vi "Touch and Limit controller.vi"(3 "error in (no error)":errorcluster) -> (0 "error out":errorcluster={"status"=TRUE, "code"=1172, "source"="Error calling method Aerotech.A3200.LabVIEW.DiagPacketPoller.Retrieve, (System.Reflection.TargetInvocationException: Exception has been thrown by the target of an invocation.\n\tInner Exception: System.NullReferenceException: Object reference not set to an instance of an object.) <append><b>System.NullReferenceException</b> in RetrieveDiagPacket.vi->Faults and Position data.vi->Aerotech Controller (main).vi"}, 1 "Limit Reached":bool, 2 "Touching":bool)   [LabVIEW 2011]
uses:
  <vilib>/DAQmx/read.llb/DAQmx Read (Digital Bool 1Line 1Point).vi
  <vilib>/DAQmx/create/channels.llb/DAQmx Create Channel (DI-Digital Input).vi
  <vilib>/DAQmx/miscellaneous.llb/DAQmx Fill In Error Info.vi
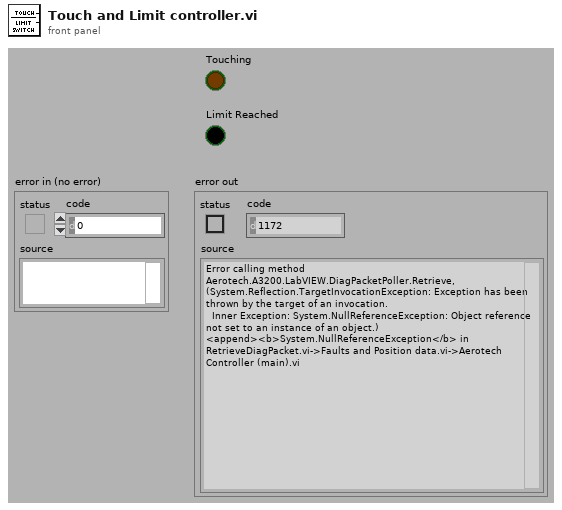
[diagram p1: front panel]
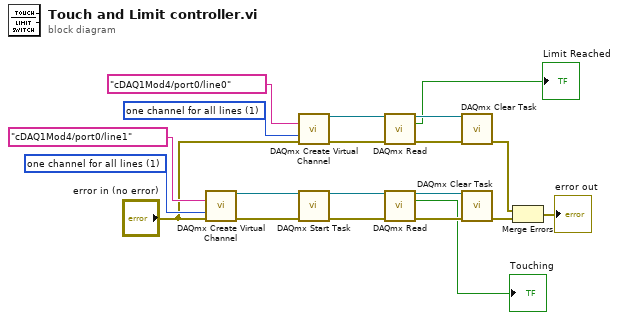
[diagram p0: block diagram]
diagram:
  w11 = 1 items=["one channel for each line", "one channel for all lines"] ("line grouping")
  w19 = 1 items=["one channel for each line", "one channel for all lines"] ("line grouping")
  n1 = call-poly <vilib>:"DAQmx Create Virtual Channel.vi"("lines"=tag "cDAQ1Mod4/port0/line1" ("Lines 2"), "line grouping"=w19, "error in"="error in (no error)") -> ("task out"=w18:refnum<k21>, "error out"=w17:errorcluster)  [unwired: 2 in, 9 out]
  n2 = call-poly <vilib>:"DAQmx Create Virtual Channel.vi"("lines"=tag "cDAQ1Mod4/port0/line0" ("Lines 2"), "line grouping"=w11, "error in"="error in (no error)") -> ("task out"=w9:refnum<k21>, "error out"=w8:errorcluster)  [unwired: 2 in, 9 out]
  n3 = call <vilib>:"DAQmx Start Task.vi"("task/channels in"=w18, "error in"=w17) -> ("task out"=w16:refnum<k21>, "error out"=w15:errorcluster)  [unwired: 12 out]
  n4 = call-poly <vilib>:"DAQmx Read.vi"("task/channels in"=w9, "error in"=w8) -> ("task out"=w7:refnum<k21>, "data"=→"Limit Reached":bool, "error out"=w6:errorcluster)  [unwired: 11 out]
  n5 = call-poly <vilib>:"DAQmx Read.vi"("task/channels in"=w16, "error in"=w15) -> ("task out"=w14:refnum<k21>, "data"=→"Touching":bool, "error out"=w13:errorcluster)  [unwired: 11 out]
  n6 = call <vilib>:"DAQmx Clear Task.vi"("task in"=w7, "error in"=w6) -> ("error out"=w5:errorcluster)  [unwired: 13 out]
  n7 = call <vilib>:"DAQmx Clear Task.vi"("task in"=w14, "error in"=w13) -> ("error out"=w4:errorcluster)  [unwired: 13 out]
  n8 = Merge Errors(w5, w4) -> (→"error out":errorcluster)
